vi "ReadSpectrometerFile.vi"(8 "error in (no error)":errorcluster, 11 "FileNameAndPath":path caption="Path") -> (0 "error out":errorcluster, 3 "Spectrometer Result":cluster{"Array":dbl[], "Array":dbl[]})   [LabVIEW 2017]
panel:
  out "text":string[](array[string])
  out "Raman Spectra from FHR":cluster{"Array":dbl[], "Array":dbl[]}(graph) caption="XY Graph - dark"
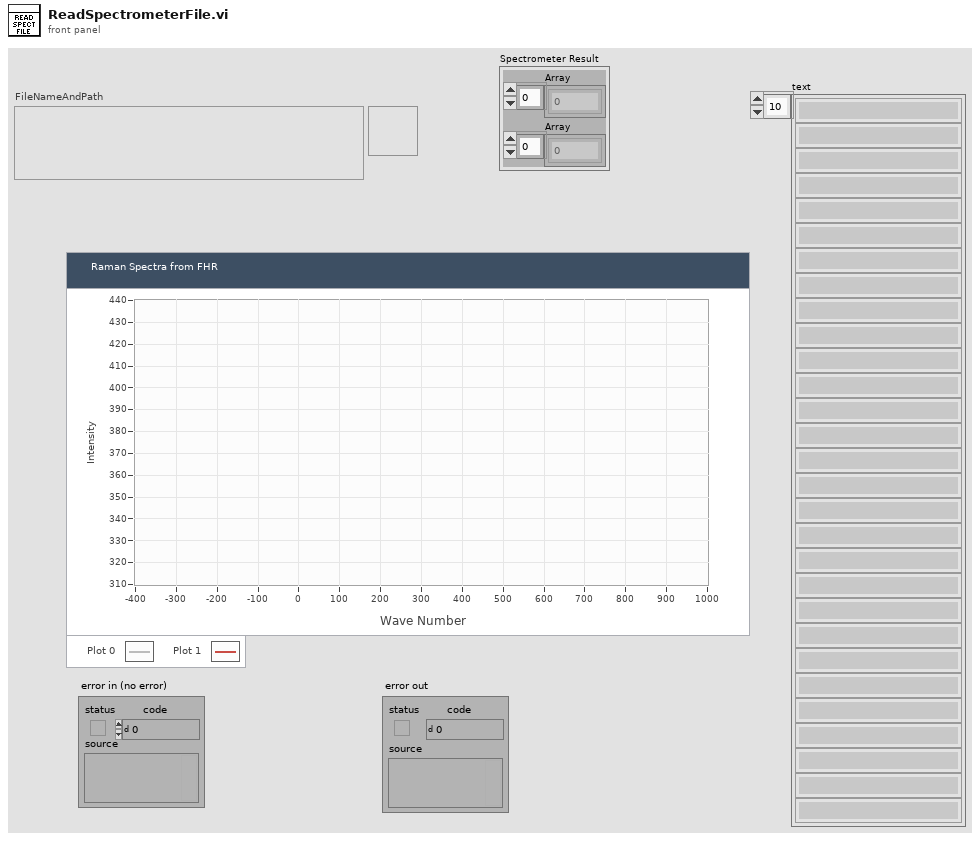
[diagram p1: front panel]
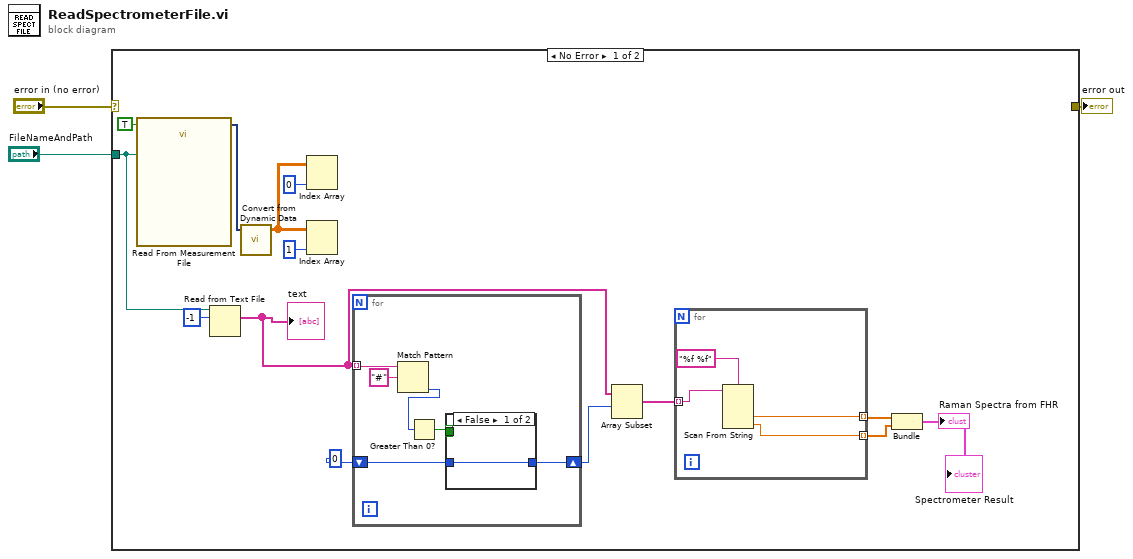
[diagram p0: block diagram]
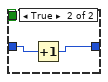
[diagram p2: hidden frame]
diagram:
  n1 = case shown="No Error" "error in (no error)" {
    selector: "error in (no error)" -> [_ w31]
    tunnel: [_ w31] -> w2
    tunnel: "FileNameAndPath" -> [w11 _]
    frame No Error {
      n2 = call "Read From Measurement File"("Filename"=w11, "Reset"=TRUE) -> ("Signals"=w17:dynamicdata)  [unwired: 4 in, 5 out]
      n3 = Read from Text File(file (use dialog)=w11, count=-1) -> (text=w7:string[])  [unwired: 2 in, 3 out]
      "text" <- w7
      n4 = call "Convert from Dynamic Data"("Dynamic Data Type"=w17) -> ("Array"=w16:dbl[][])  [unwired: 3 in]
      n5 = Index Array(array=w16, index (col)=0 ("disabled index (col)")) -> ()  [unwired: 1 in, 1 out]
      n6 = Index Array(array=w16, index (col)=1 ("disabled index (col)")) -> ()  [unwired: 1 in, 1 out]
      n7 = for {
        tunnel: w7 -> [w27] mode=indexing
        shift-right: [w22] -> w8
        shift-left: 0 -> [w23]
        n8 = Match Pattern(string=w27, regular expression="#") -> (offset past match=w25:i32)  [unwired: 1 in, 3 out]
        n9 = Greater Than 0?(x=w25) -> (x > 0?=w24:bool)
        n10 = case shown="False" w24 {
          tunnel: w24 -> [_ _]
          tunnel: w23 -> [w28 w30]
          tunnel: [w28 w29] -> w22
          frame False {
          }
          frame True {
            n11 = Increment(x=w30) -> (x+1=w29:i32)
          }
        }
      }
      n12 = Array Subset(array=w7, index=w8) -> (w6:string[])  [unwired: 1 in]
      n13 = for {
        tunnel: w6 -> [w21] mode=indexing
        tunnel: [w19] -> w5 mode=indexing
        tunnel: [w18] -> w4 mode=indexing
        n14 = Scan From String(format string="%f %f", input string=w21) -> (output 1=w19:dbl, output 2=w18:dbl)  [unwired: 4 in, 3 out]
      }
      n15 = Bundle(w5, w4) -> (→"Raman Spectra from FHR" →"Spectrometer Result":cluster{dbl[], dbl[]})  [unwired: 1 in]
    }
    frame Error {
    }
  }
  "error out" <- w2
